vi "C400 Example.vi"() -> ()   [LabVIEW 2017]
panel:
  in  "phase":dbl format="%.2p"
  in  "frequency":dbl=1.0 format="%0.2p"
  in  "amplitude":dbl=10.0 format="%0.2p"
  in  "signal type":T1(ring)
  in  "offset":dbl format="%0.2p"
  in  "Stop Waveform":bool
  in  "Start Waveform":bool
  in  "Run Chart":bool
  out "Sensor Reading Waveform Chart":dbl(graph)=-15.449458025852254
  out "Ch1 Position Units":string
  out "Ch1Range":i32
  in  "Read Sensor":bool
  out "Ch1 Sensor Value":dbl format="%.3f"
  out "Serial Number Array":string[](array[string])
  out "FT_Status":u32(ring) items=["FT_OK", "FT_INVALID_HANDLE", "FT_DEVICE_NOT_FOUND", "FT_DEVICE_NOT_OPENED", "FT_IO_ERROR", "FT_INSUFFICIENT_RESOURCES", "FT_INVALID_PARAMETER", "FT_INVALID_BAUD_RATE", "FT_DEVICE_NOT_OPENED_FOR_ERASE", "FT_DEVICE_NOT_OPENED_FOR_WRITE", "FT_FAILED_TO_WRITE_DEVICE", "FT_EEPROM_READ_FAILED", "FT_EEPROM_WRITE_FAILED", "FT_EEPROM_ERASE_FAILED", "FT_EEPROM_NOT_PRESENT", "FT_EEPROM_NOT_PROGRAMMED", "FT_INVALID_ARGS", "FT_NOT_SUPPORTED", "FT_OTHER_ERROR"]
  in  "Ch1 Position Cmd":dbl format="%.3f"
  in  "Connect":bool
  in  "Stop Button":bool
  in  "Listbox":i32(listbox)=-1
  in  "Handle":i32
  # "Waveform Controls"
  # "FT_Status displays the error type if an\nFTDI USB function did not execute properly."
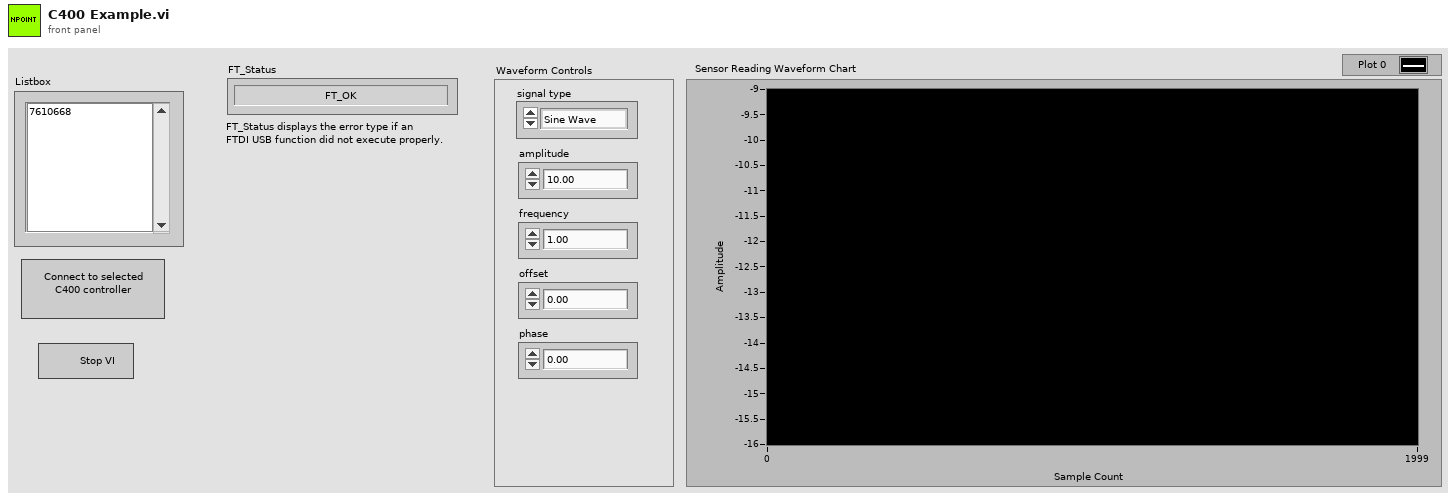
[diagram p1: front panel]
types:
  T1 = enum16{"Sine Wave", "Triangle Wave", "Square Wave", "Sawtooth Wave"}
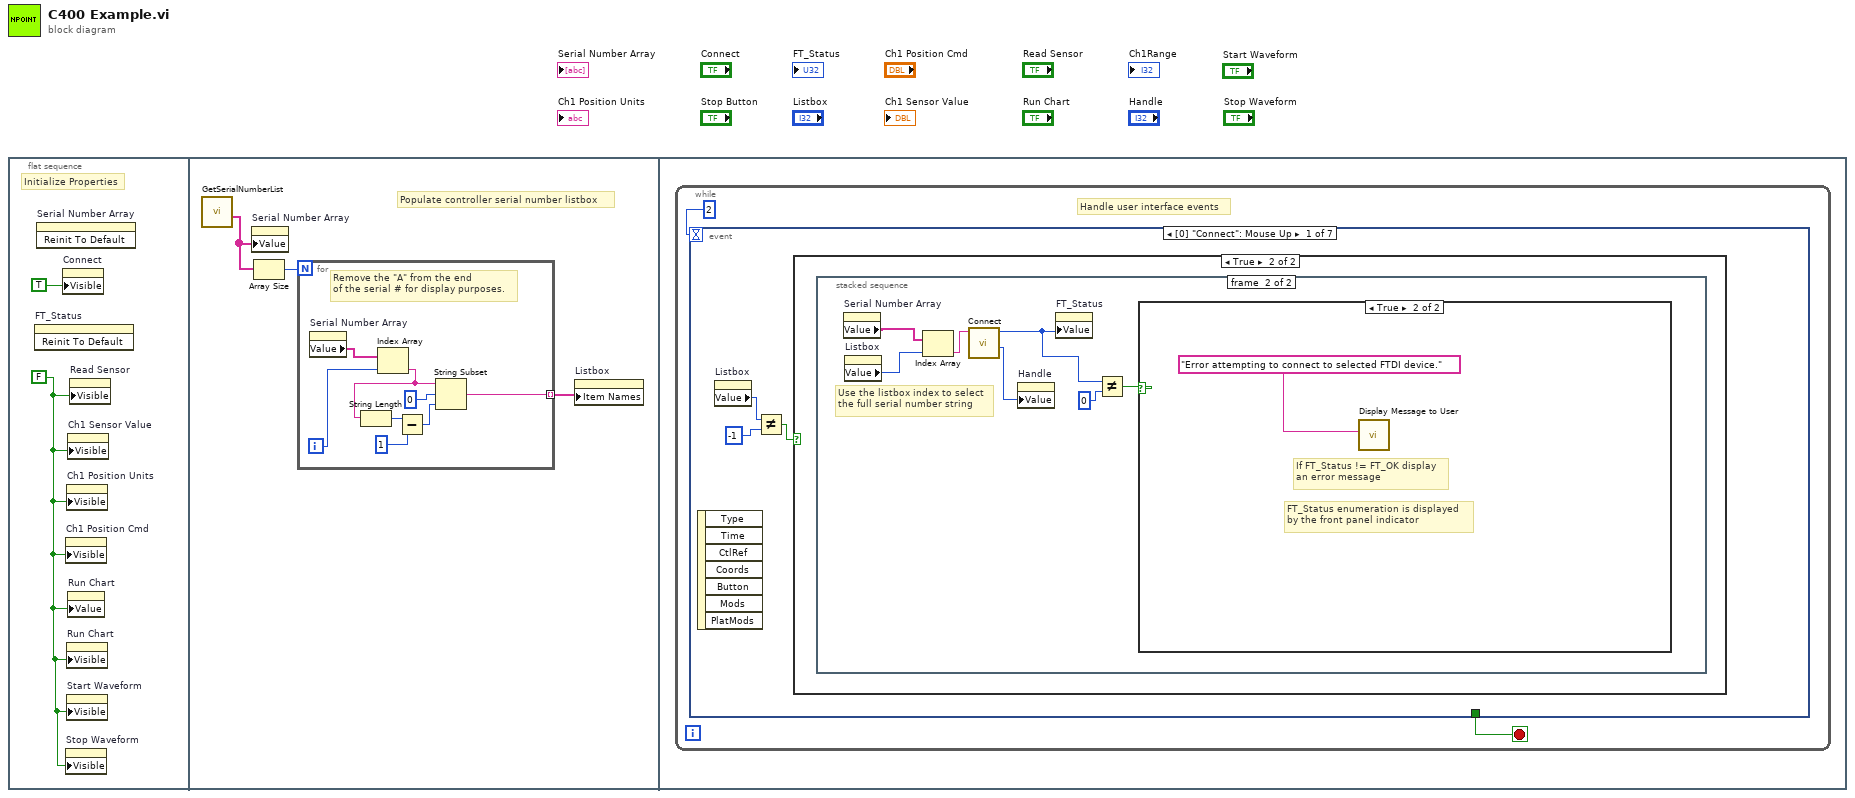
[diagram p0: block diagram]
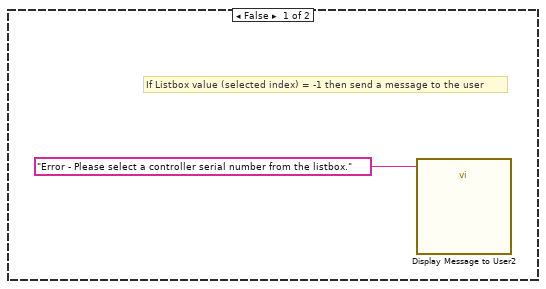
[diagram p2: hidden frame]
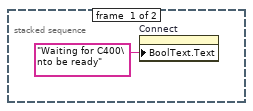
[diagram p3: hidden frame]
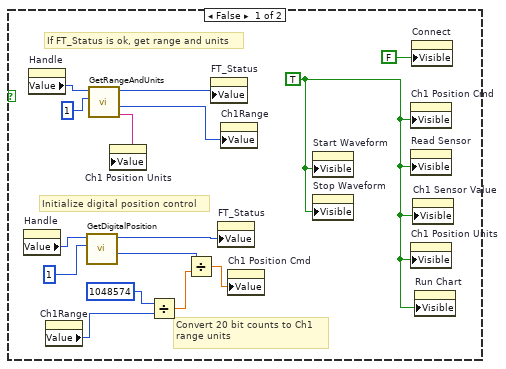
[diagram p4: hidden frame]
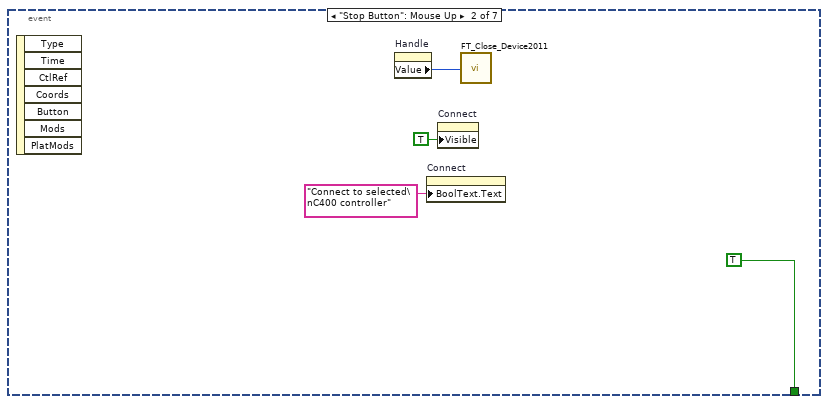
[diagram p5: hidden frame]
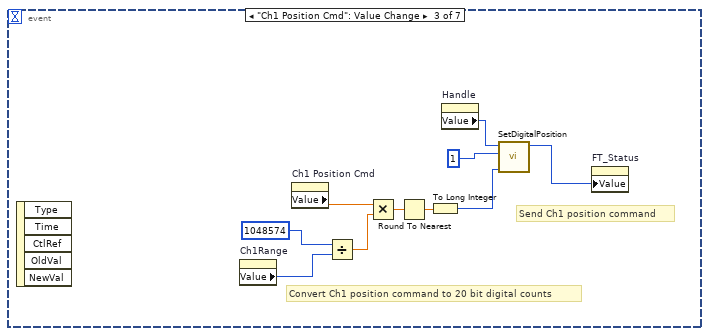
[diagram p6: hidden frame]
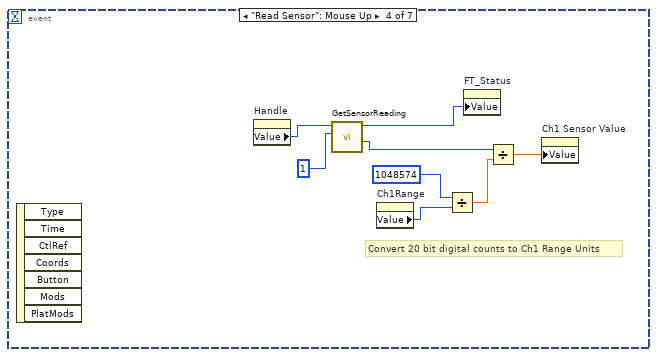
[diagram p7: hidden frame]
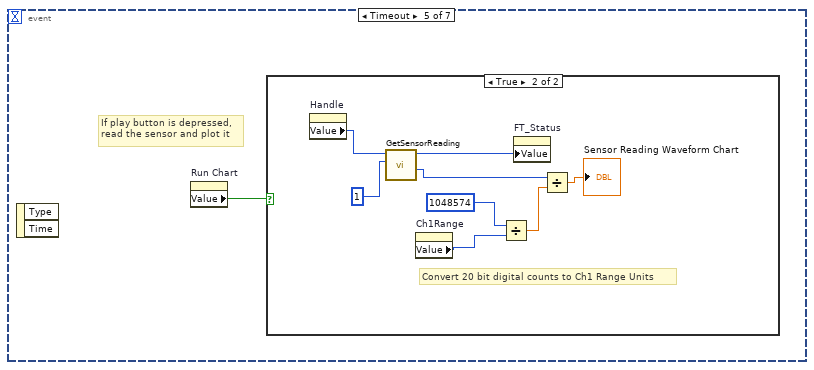
[diagram p8: hidden frame]
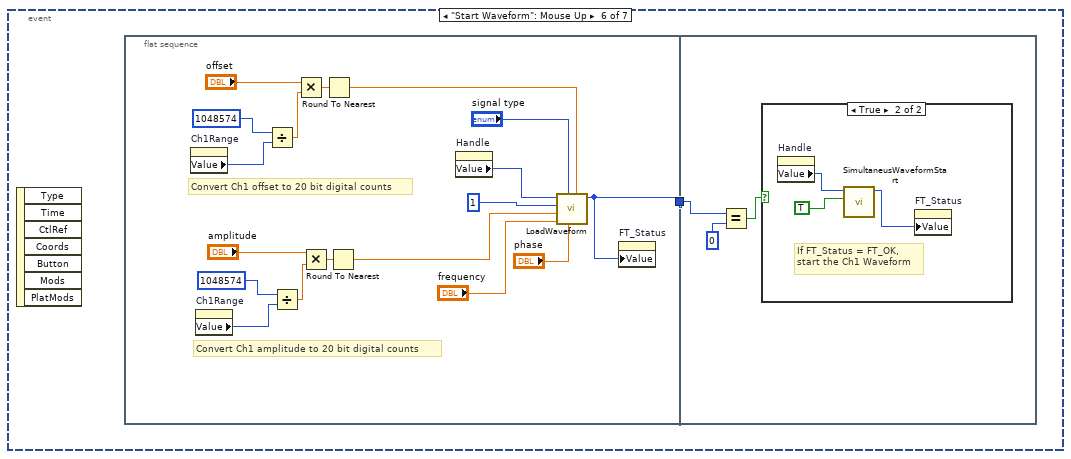
[diagram p10: hidden frame]
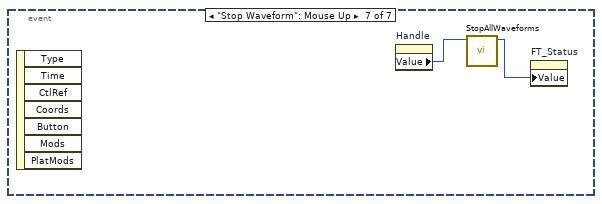
[diagram p12: hidden frame]
diagram:
  n1 = flat-sequence {
    frame #0 {
      w1 = FALSE ("Visible")
      # "Initialize Properties"
      n2 = invoke on="FT_Status" class="Ring (strict)" method="Reinit To Default"() -> ()  [unwired: 3 in, 3 out]
      n3 = invoke on="Serial Number Array" class="Arr (strict)" method="Reinit To Default"() -> ()  [unwired: 3 in, 3 out]
      n4 = property on="Connect" class="Bool (strict)"("Visible"=TRUE) -> ()  [unwired: 2 in, 2 out]
      n5 = property on="Ch1 Position Cmd" class="DigNum (strict)"("Visible"=w1) -> ()  [unwired: 2 in, 2 out]
      n6 = property on="Stop Waveform" class="Bool (strict)"("Visible"=w1) -> ()  [unwired: 2 in, 2 out]
      n7 = property on="Ch1 Position Units" class="Str"("Visible"=w1) -> ()  [unwired: 2 in, 2 out]
      n8 = property on="Run Chart" class="Bool (strict)"("Visible"=w1) -> ()  [unwired: 2 in, 2 out]
      n9 = property on="Start Waveform" class="Bool (strict)"("Visible"=w1) -> ()  [unwired: 2 in, 2 out]
      n10 = property on="Ch1 Sensor Value" class="DigNum (strict)"("Visible"=w1) -> ()  [unwired: 2 in, 2 out]
      n11 = property on="Run Chart" class="Bool (strict)"("Value"=w1) -> ()  [unwired: 2 in, 2 out]
      n12 = property on="Read Sensor" class="Bool (strict)"("Visible"=w1) -> ()  [unwired: 2 in, 2 out]
    }
    frame #1 {
      # "Populate controller serial number listbox"
      n13 = call "GetSerialNumberList.vi"() -> ("C400 Serial Number Array"=w4:string[])  [unwired: 11 in]
      n14 = property on="Serial Number Array" class="Arr (strict)"("Value"=w4) -> ()  [unwired: 2 in, 2 out]
      n15 = Array Size(array=w4) -> (size(s)=w5:i32)
      n16 = for {
        N: w5 -> [_]
        tunnel: [w6] -> w3 mode=indexing
        i -> [w13]
        # "Remove the \"A\" from the end\nof the serial # for display purposes."
        n17 = property on="Serial Number Array" class="Arr (strict)"() -> ("Value"=w9:string[])  [unwired: 2 in, 2 out]
        n18 = Index Array(array=w9, index=w13) -> (element=w7:string)
        n19 = String Length(string=w7) -> (length=w11:i32)
        n20 = Subtract(x=w11, y=1) -> (x-y=w8:i32)
        n21 = String Subset(string=w7, offset (0)=0, length (rest)=w8) -> (substring=w6:string)
      }
      n22 = property on="Listbox" class="LstBox (strict)"("Item Names"=w3) -> ()  [unwired: 2 in, 2 out]
    }
    frame #2 {
      n23 = while {
        stop <- w15 stop-if-true
        # "Handle user interface events"
        n24 = event shown="[0] \"Connect\": Mouse Up" {
          selector: _ -> [_ _ _ _ _ _ _]
          dyn-events: _ -> [_ _ _ _ _ _ _]
          timeout: 2 -> [_ _ _ _ _ _ _]
          tunnel: [_ TRUE _ _ _ _ _] -> w15
          event "Connect": Mouse Up {
            n25 = event-data() -> ()  [unwired: 1 in, 7 out]
            n26 = property on="Listbox" class="LstBox (strict)"() -> ("Value"=w17:i32)  [unwired: 2 in, 2 out]
            n27 = Not Equal?(x=w17, y=-1) -> (x != y?=w18:bool)
            n28 = case shown="True" w18 {
              frame False {
                # "If Listbox value (selected index) = -1 then send a message to the user"
                n29 = call "Display Message to User2"("Message"="Error - Please select a controller serial number from the listbox.") -> ()  [unwired: 9 in, 2 out]
              }
              frame True {
                n30 = stacked-sequence {
                  frame #0 {
                    n31 = property on="Connect" class="Bool (strict)"("BoolText.Text"="Waiting for C400\nto be ready" ("Boolean Text.Text")) -> ()  [unwired: 2 in, 2 out]
                  }
                  frame #1 {
                    # "Use the listbox index to select\nthe full serial number string"
                    n32 = property on="Serial Number Array" class="Arr (strict)"() -> ("Value"=w25:string[])  [unwired: 2 in, 2 out]
                    n33 = property on="Listbox" class="LstBox (strict)"() -> ("Value"=w24:i32)  [unwired: 2 in, 2 out]
                    n34 = Index Array(array=w25, index=w24) -> (element=w23:string)
                    n35 = call "Connect.vi"("Device Serial Number"=w23) -> ("Handle"=w21:u32, "FT_Status"=w22:u32)  [unwired: 9 in]
                    n36 = property on="Handle" class="DigNum (strict)"("Value"=w21) -> ()  [unwired: 2 in, 2 out]
                    n37 = property on="FT_Status" class="Ring (strict)"("Value"=w22) -> ()  [unwired: 2 in, 2 out]
                    n38 = Not Equal?(x=w22, y=u32 0) -> (x != y?=w26:bool)
                    n39 = case shown="True" w26 {
                      frame False {
                        w28 = TRUE ("Visible")
                        # "Convert 20 bit counts to Ch1\nrange units"
                        # "Initialize digital position control"
                        # "If FT_Status is ok, get range and units"
                        n40 = property on="Handle" class="DigNum (strict)"() -> ("Value"=w39:i32)  [unwired: 2 in, 2 out]
                        n41 = property on="Handle" class="DigNum (strict)"() -> ("Value"=w42:i32)  [unwired: 2 in, 2 out]
                        n42 = property on="Ch1Range" class="DigNum (strict)"() -> ("Value"=w32:i32)  [unwired: 2 in, 2 out]
                        n43 = call "GetDigitalPosition.vi"("Handle"=w39, "Controller Channel"=1) -> ("FT_Status"=w37:u32, "Position"=w31:i32)  [unwired: 7 in]
                        n44 = call "GetRangeAndUnits.vi"("Handle"=w42, "Controller Channel"=1) -> ("FT_Status"=w36:u32, "Range"=w40:i32, "Range Units"=w35:string)  [unwired: 6 in]
                        n45 = property on="Ch1 Position Units" class="Str"("Value"=w35) -> ()  [unwired: 2 in, 2 out]
                        n46 = Divide(x=1048574, y=w32) -> (x/y=w33:dbl)
                        n47 = Divide(x=w31, y=w33) -> (x/y=w30:dbl)
                        n48 = property on="FT_Status" class="Ring (strict)"("Value"=w36) -> ()  [unwired: 2 in, 2 out]
                        n49 = property on="FT_Status" class="Ring (strict)"("Value"=w37) -> ()  [unwired: 2 in, 2 out]
                        n50 = property on="Ch1Range" class="DigNum (strict)"("Value"=w40) -> ()  [unwired: 2 in, 2 out]
                        n51 = property on="Ch1 Position Cmd" class="DigNum (strict)"("Value"=w30) -> ()  [unwired: 2 in, 2 out]
                        n52 = property on="Start Waveform" class="Bool (strict)"("Visible"=w28) -> ()  [unwired: 2 in, 2 out]
                        n53 = property on="Stop Waveform" class="Bool (strict)"("Visible"=w28) -> ()  [unwired: 2 in, 2 out]
                        n54 = property on="Ch1 Position Cmd" class="DigNum (strict)"("Visible"=w28) -> ()  [unwired: 2 in, 2 out]
                        n55 = property on="Read Sensor" class="Bool (strict)"("Visible"=w28) -> ()  [unwired: 2 in, 2 out]
                        n56 = property on="Ch1 Position Units" class="Str"("Visible"=w28) -> ()  [unwired: 2 in, 2 out]
                        n57 = property on="Connect" class="Bool (strict)"("Visible"=FALSE) -> ()  [unwired: 2 in, 2 out]
                        n58 = property on="Ch1 Sensor Value" class="DigNum (strict)"("Visible"=w28) -> ()  [unwired: 2 in, 2 out]
                        n59 = property on="Run Chart" class="Bool (strict)"("Visible"=w28) -> ()  [unwired: 2 in, 2 out]
                      }
                      frame True {
                        # "FT_Status enumeration is displayed\nby the front panel indicator"
                        # "If FT_Status != FT_OK display\nan error message"
                        n60 = call "Display Message to User"("Message"="Error attempting to connect to selected FTDI device.") -> ()  [unwired: 9 in, 2 out]
                      }
                    }
                  }
                }
              }
            }
          }
          event "Stop Button": Mouse Up {
            n61 = event-data() -> ()  [unwired: 1 in, 7 out]
            n62 = property on="Handle" class="DigNum (strict)"() -> ("Value"=w46:i32)  [unwired: 2 in, 2 out]
            n63 = property on="Connect" class="Bool (strict)"("BoolText.Text"="Connect to selected\nC400 controller" ("Boolean Text.Text")) -> ()  [unwired: 2 in, 2 out]
            n64 = property on="Connect" class="Bool (strict)"("Visible"=TRUE) -> ()  [unwired: 2 in, 2 out]
            n65 = call "FT_Close_Device2011.vi"("Handle"=w46) -> ()  [unwired: 1 out]
          }
          event "Ch1 Position Cmd": Value Change {
            # "Send Ch1 position command"
            # "Convert Ch1 position command to 20 bit digital counts"
            n66 = event-data() -> ()  [unwired: 1 in, 5 out]
            n67 = property on="Ch1Range" class="DigNum (strict)"() -> ("Value"=w53:i32)  [unwired: 2 in, 2 out]
            n68 = property on="Ch1 Position Cmd" class="DigNum (strict)"() -> ("Value"=w54:dbl)  [unwired: 2 in, 2 out]
            n69 = Divide(x=1048574, y=w53) -> (x/y=w51:dbl)
            n70 = Multiply(x=w54, y=w51) -> (x*y=w50:dbl)
            n71 = Round To Nearest(number=w50) -> (nearest integer value=w49:dbl)
            n72 = To Long Integer(number=w49) -> (32bit integer=w48:i32)
            n73 = property on="Handle" class="DigNum (strict)"() -> ("Value"=w57:i32)  [unwired: 2 in, 2 out]
            n74 = call "SetDigitalPosition.vi"("Position"=w48, "Controller Channel"=1, "Handle"=w57) -> ("FT_Status"=w55:u32)  [unwired: 8 in]
            n75 = property on="FT_Status" class="Ring (strict)"("Value"=w55) -> ()  [unwired: 2 in, 2 out]
          }
          event "Read Sensor": Mouse Up {
            # "Convert 20 bit digital counts to Ch1 Range Units"
            n76 = event-data() -> ()  [unwired: 1 in, 7 out]
            n77 = property on="Handle" class="DigNum (strict)"() -> ("Value"=w65:i32)  [unwired: 2 in, 2 out]
            n78 = call "GetSensorReading.vi"("Handle"=w65, "Controller Channel"=1) -> ("FT_Status"=w63:u32, "Sensor Reading"=w60:i32)  [unwired: 7 in]
            n79 = property on="Ch1Range" class="DigNum (strict)"() -> ("Value"=w62:i32)  [unwired: 2 in, 2 out]
            n80 = Divide(x=1048574, y=w62) -> (x/y=w59:dbl)
            n81 = property on="FT_Status" class="Ring (strict)"("Value"=w63) -> ()  [unwired: 2 in, 2 out]
            n82 = Divide(x=w60, y=w59) -> (x/y=w58:dbl)
            n83 = property on="Ch1 Sensor Value" class="DigNum (strict)"("Value"=w58) -> ()  [unwired: 2 in, 2 out]
          }
          event Timeout {
            # "If play button is depressed,\nread the sensor and plot it"
            n84 = event-data() -> ()  [unwired: 1 in, 2 out]
            n85 = property on="Run Chart" class="Bool (strict)"() -> ("Value"=w66:bool)  [unwired: 2 in, 2 out]
            n86 = case shown="True" w66 {
              frame False {
              }
              frame True {
                # "Convert 20 bit digital counts to Ch1 Range Units"
                n87 = property on="Handle" class="DigNum (strict)"() -> ("Value"=w69:i32)  [unwired: 2 in, 2 out]
                n88 = call "GetSensorReading.vi"("Handle"=w69, "Controller Channel"=1) -> ("FT_Status"=w68:u32, "Sensor Reading"=w72:i32)  [unwired: 7 in]
                n89 = property on="Ch1Range" class="DigNum (strict)"() -> ("Value"=w70:i32)  [unwired: 2 in, 2 out]
                n90 = Divide(x=1048574, y=w70) -> (x/y=w71:dbl)
                n91 = property on="FT_Status" class="Ring (strict)"("Value"=w68) -> ()  [unwired: 2 in, 2 out]
                n92 = Divide(x=w72, y=w71) -> (x/y=→"Sensor Reading Waveform Chart":dbl)
              }
            }
          }
          event "Start Waveform": Mouse Up {
            n93 = event-data() -> ()  [unwired: 1 in, 7 out]
            n94 = flat-sequence {
              tunnel: [w92] -> w75
              tunnel: w75 -> [w96]
              frame #0 {
                # "Convert Ch1 offset to 20 bit digital counts"
                # "Convert Ch1 amplitude to 20 bit digital counts"
                n95 = property on="Ch1Range" class="DigNum (strict)"() -> ("Value"=w79:i32)  [unwired: 2 in, 2 out]
                n96 = property on="Ch1Range" class="DigNum (strict)"() -> ("Value"=w87:i32)  [unwired: 2 in, 2 out]
                n97 = Divide(x=1048574, y=w79) -> (x/y=w77:dbl)
                n98 = Divide(x=1048574, y=w87) -> (x/y=w85:dbl)
                n99 = Multiply(x="offset", y=w77) -> (x*y=w81:dbl)
                n100 = Multiply(x="amplitude", y=w85) -> (x*y=w84:dbl)
                n101 = Round To Nearest(number=w81) -> (nearest integer value=w76:dbl)
                n102 = Round To Nearest(number=w84) -> (nearest integer value=w82:dbl)
                n103 = property on="Handle" class="DigNum (strict)"() -> ("Value"=w93:i32)  [unwired: 2 in, 2 out]
                n104 = call "LoadWaveform.vi"("offset"=w76, "phase"="phase", "signal type"="signal type", "frequency"="frequency", "amplitude"=w82, "Channel"=1 ("Controller Channel"), "Handle"=w93) -> ("FT_Status"=w92:u32)  [unwired: 4 in]
                n105 = property on="FT_Status" class="Ring (strict)"("Value"=w92) -> ()  [unwired: 2 in, 2 out]
              }
              frame #1 {
                n106 = Equal?(x=w96, y=u32 0) -> (x = y?=w94:bool)
                n107 = case shown="True" w94 {
                  frame False {
                  }
                  frame True {
                    # "If FT_Status = FT_OK,\nstart the Ch1 Waveform"
                    n108 = property on="Handle" class="DigNum (strict)"() -> ("Value"=w99:i32)  [unwired: 2 in, 2 out]
                    n109 = call "SimultaneusWaveformStart.vi"("Ch1Start"=TRUE, "Handle"=w99) -> ("FT_Status"=w97:u32)  [unwired: 9 in]
                    n110 = property on="FT_Status" class="Ring (strict)"("Value"=w97) -> ()  [unwired: 2 in, 2 out]
                  }
                }
              }
            }
          }
          event "Stop Waveform": Mouse Up {
            n111 = event-data() -> ()  [unwired: 1 in, 7 out]
            n112 = property on="Handle" class="DigNum (strict)"() -> ("Value"=w101:i32)  [unwired: 2 in, 2 out]
            n113 = call "StopAllWaveforms.vi"("Handle"=w101) -> ("FT_Status"=w100:u32)  [unwired: 10 in]
            n114 = property on="FT_Status" class="Ring (strict)"("Value"=w100) -> ()  [unwired: 2 in, 2 out]
          }
        }
      }
    }
  }
